vi "gentec-M-Link.Flush Buffer.vi"(0 "VISA resource(In)":refnum<visa-resource-name>, 5 "error in (no error)":errorcluster) -> (14 "VISA resource (out)":refnum<visa-resource-name>, 17 "Success":bool, 19 "error out":errorcluster)   [LabVIEW 2014, in "gentec-M-Link - Driver.lvlib"]
doc: "This VI calls a VISA \"Flush I/O Buffer\"."
uses:
  gentec-M-Link - Driver.lvlib
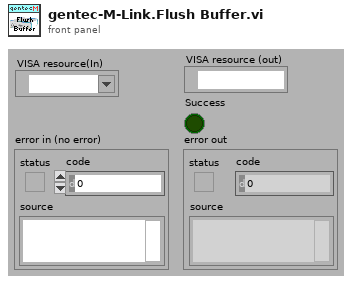
[diagram p1: front panel]
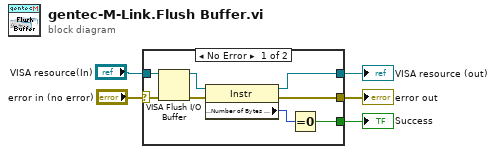
[diagram p0: block diagram]
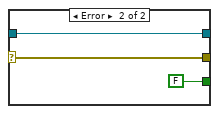
[diagram p2: hidden frame]
diagram:
  n1 = case shown="No Error" "error in (no error)" {
    selector: "error in (no error)" -> [w10 w16]
    tunnel: [w12 w16] -> w4
    tunnel: "VISA resource(In)" -> [w9 w14]
    tunnel: [w7 FALSE] -> w2
    tunnel: [w6 w14] -> w1
    frame No Error {
      n2 = VISA Flush I/O Buffer(VISA resource name=w9, error in (no error)=w10) -> (VISA resource name out=w13:refnum<visa-resource-name>, error out=w11:errorcluster)  [unwired: 1 in]
      n3 = property class="Instr"(reference=w13, error in=w11) -> (reference out=w6:refnum<visa-resource-name>, error out=w12:errorcluster, "Serial Settings:Number of Bytes at Serial Port"=w8:u32)
      n4 = Equal To 0?(x=w8) -> (x = 0?=w7:bool)
    }
    frame Error {
    }
  }
  "error out" <- w4
  "Success" <- w2
  "VISA resource (out)" <- w1
